vi "Bang-Bang Control.vi"(7 "Output Range":T1={"Maximum"=1.0, "Minimum (Probably 0)"=0.0}, 9 "Deadband Size":dbl=1.0, 10 "Process Variable":dbl(slide) scale=0.0..10.0, 11 "Setpoint":dbl) -> (3 "Output":dbl)   [LabVIEW 2012]
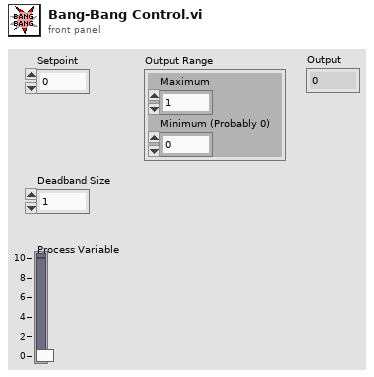
[diagram p1: front panel]
types:
  T1 = cluster{"Maximum":dbl, "Minimum (Probably 0)":dbl}
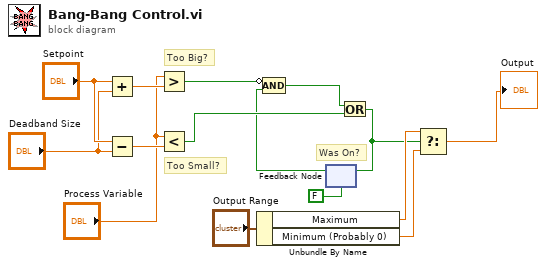
[diagram p0: block diagram]
diagram:
  # "Was On?"
  # "Too Small?"
  # "Too Big?"
  n1 = Add(x="Setpoint", y="Deadband Size") -> (x+y=w12:dbl)
  n2 = Subtract(x="Setpoint", y="Deadband Size") -> (x-y=w11:dbl)
  n3 = Greater?(x="Process Variable", y=w12) -> (0:w5:bool)
  n4 = Less?(x="Process Variable", y=w11) -> (x < y?=w4:bool)
  n5 = Unbundle By Name("Output Range") -> ("Maximum"=w9:dbl, "Minimum (Probably 0)"=w8:dbl)
  n6 = feedback #1(FALSE) -> (w1:bool)
  n7 = Compound Arithmetic op=AND(invert w5, w1) -> (w6:bool)
  n8 = Or(x=w6, y=w4) -> (x .or. y?=w2:bool)
  n9 = feedback-in #1(w2) -> ()
  n10 = Select(t=w9, s=w2, f=w8) -> (s? t:f=→"Output":dbl)
